vi "MAIN_save_acquisition_parameters_txt.vi"(3 "TL Array":dbl[][](array[numeric]), 4 "Global parameters":T2 {"# repetitions" min=0; "Dt (s)" min=0 step=1; "Filter list" items=["ET665lp", "zet405/488/561/640m", "None", "None", "None", "None"]}, 5 "List probe Refnum":refnum<vi>, 6 "file path":path, 7 "Data":T1, 8 "error in":errorcluster, 9 "ROI list Refnum":refnum<vi>, 10 "Laser list Refnum":refnum<vi>, 11 "Data type":string) -> (0 "error out":errorcluster)   [LabVIEW 2015]
uses:
  CONTROLS/Global parameters.ctl
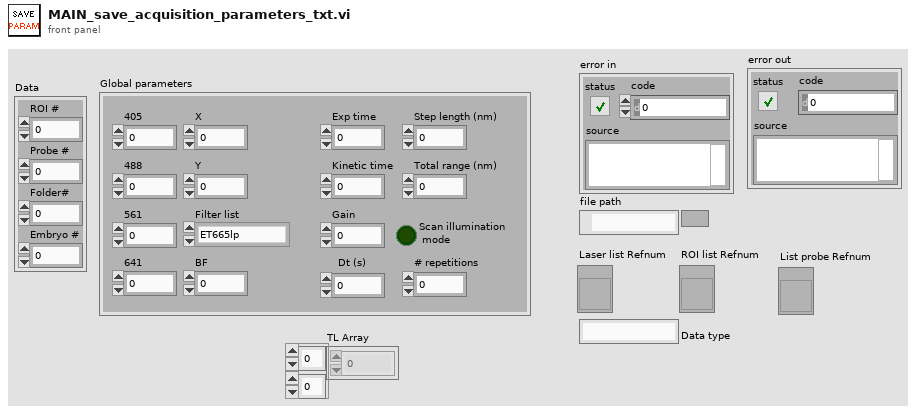
[diagram p1: front panel]
types:
  T1 = cluster{"ROI #":i32, "Probe #":i32, "Folder# ":i32, "Embryo #":i32}
  T2 = typedef "Global parameters.ctl" = cluster{"405":dbl, "488":dbl, "561":dbl, "641":dbl, "BF":dbl, "X":dbl, "Y":dbl, "Filter list":u16, "Exp time":sgl, "Kinetic time":sgl, "Gain":i32, "Step length (nm)":u32, "Total range (nm)":u32, "Scan illumination\n mode":bool, "Dt (s)":i32, "# repetitions":i32}
  T3 = enum16{"open", "replace", "create", "open or create", "replace or create", "replace or create with confirmation"}
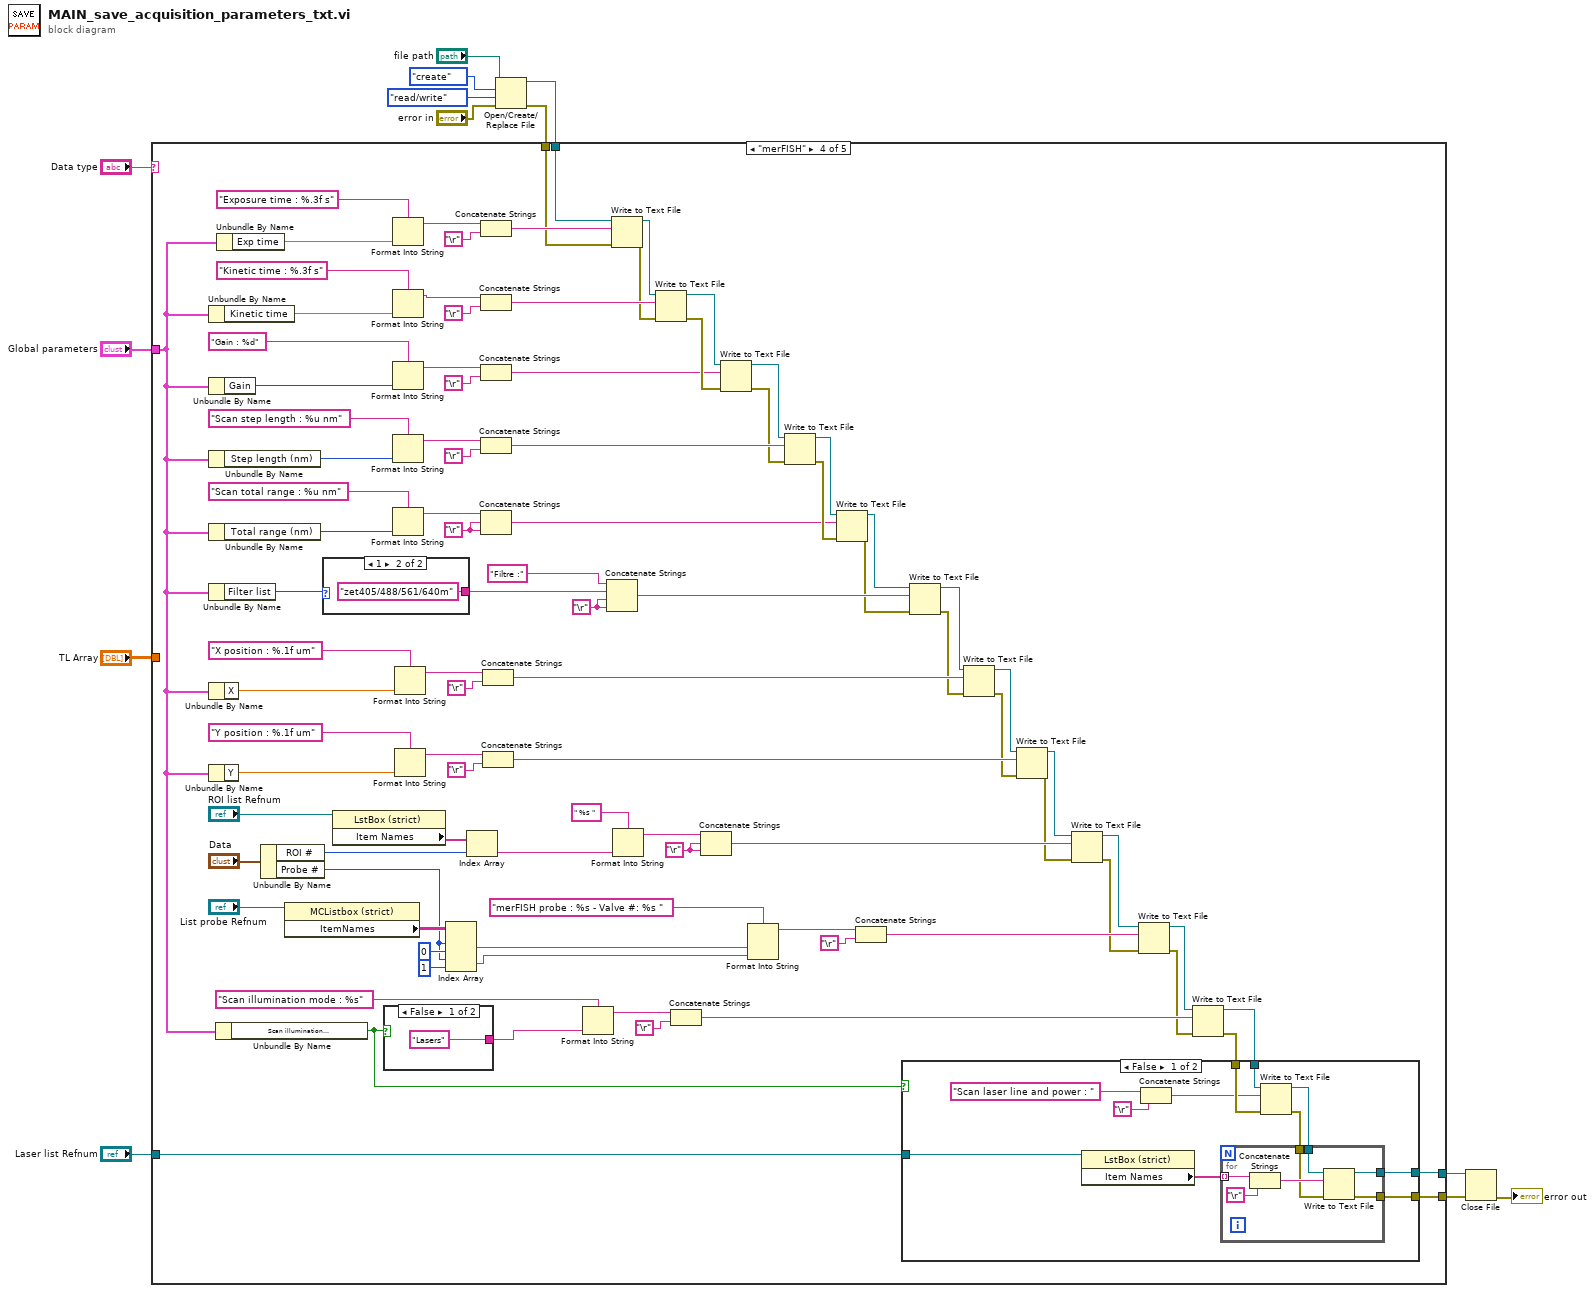
[diagram p0: block diagram]
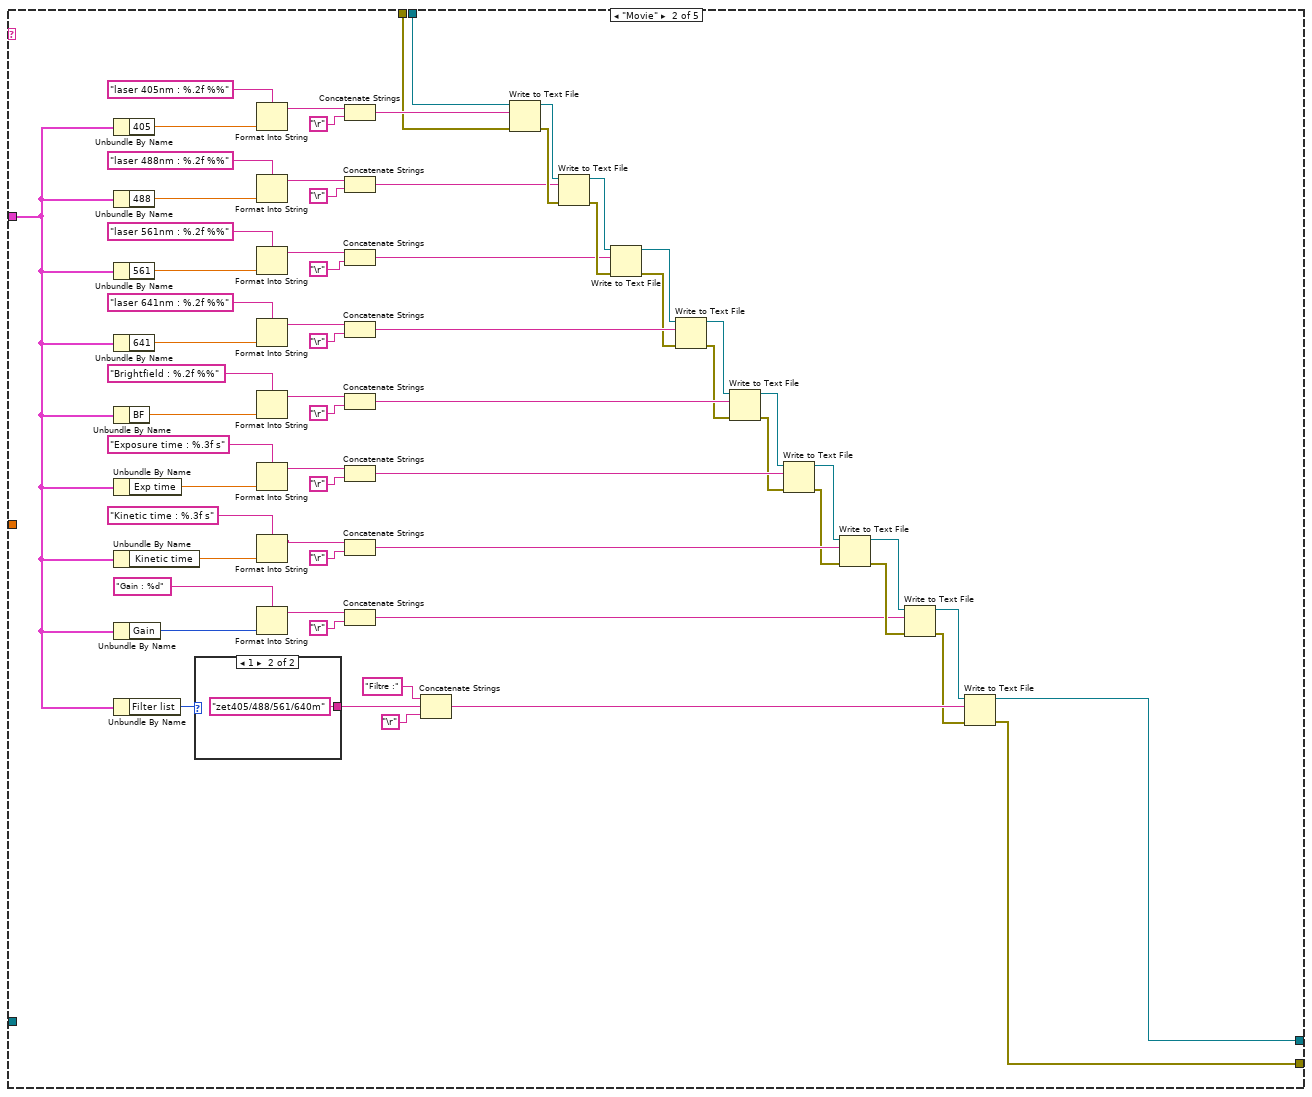
[diagram p3: hidden frame]
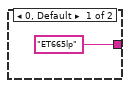
[diagram p4: hidden frame]
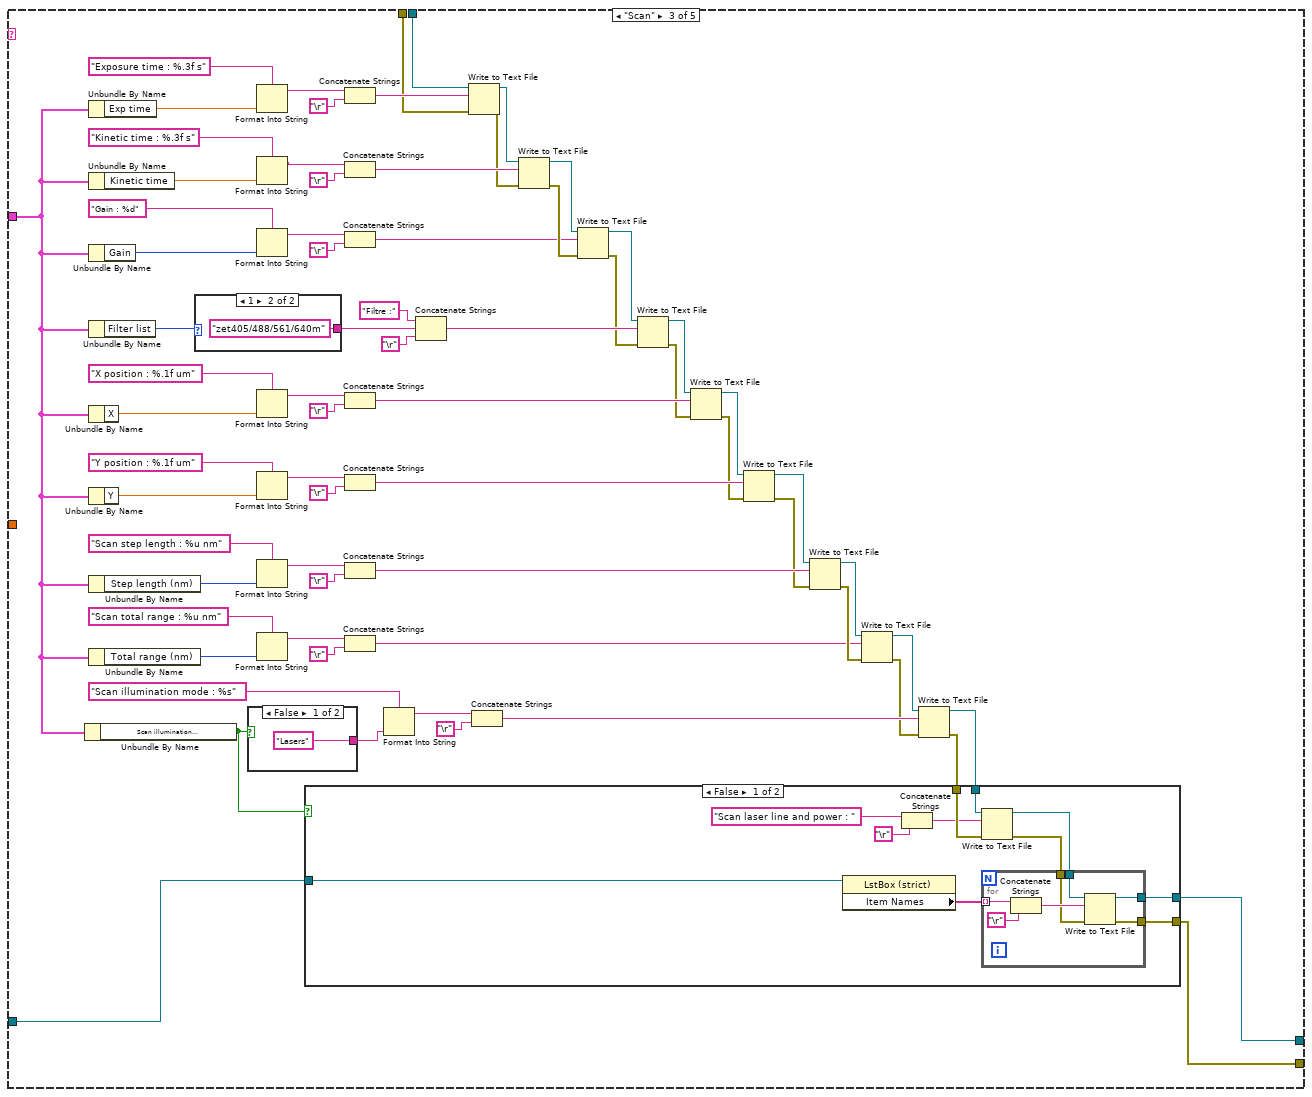
[diagram p5: hidden frame]
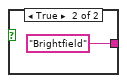
[diagram p7: hidden frame]
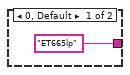
[diagram p8: hidden frame]
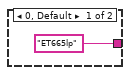
[diagram p9: hidden frame]
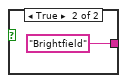
[diagram p11: hidden frame]
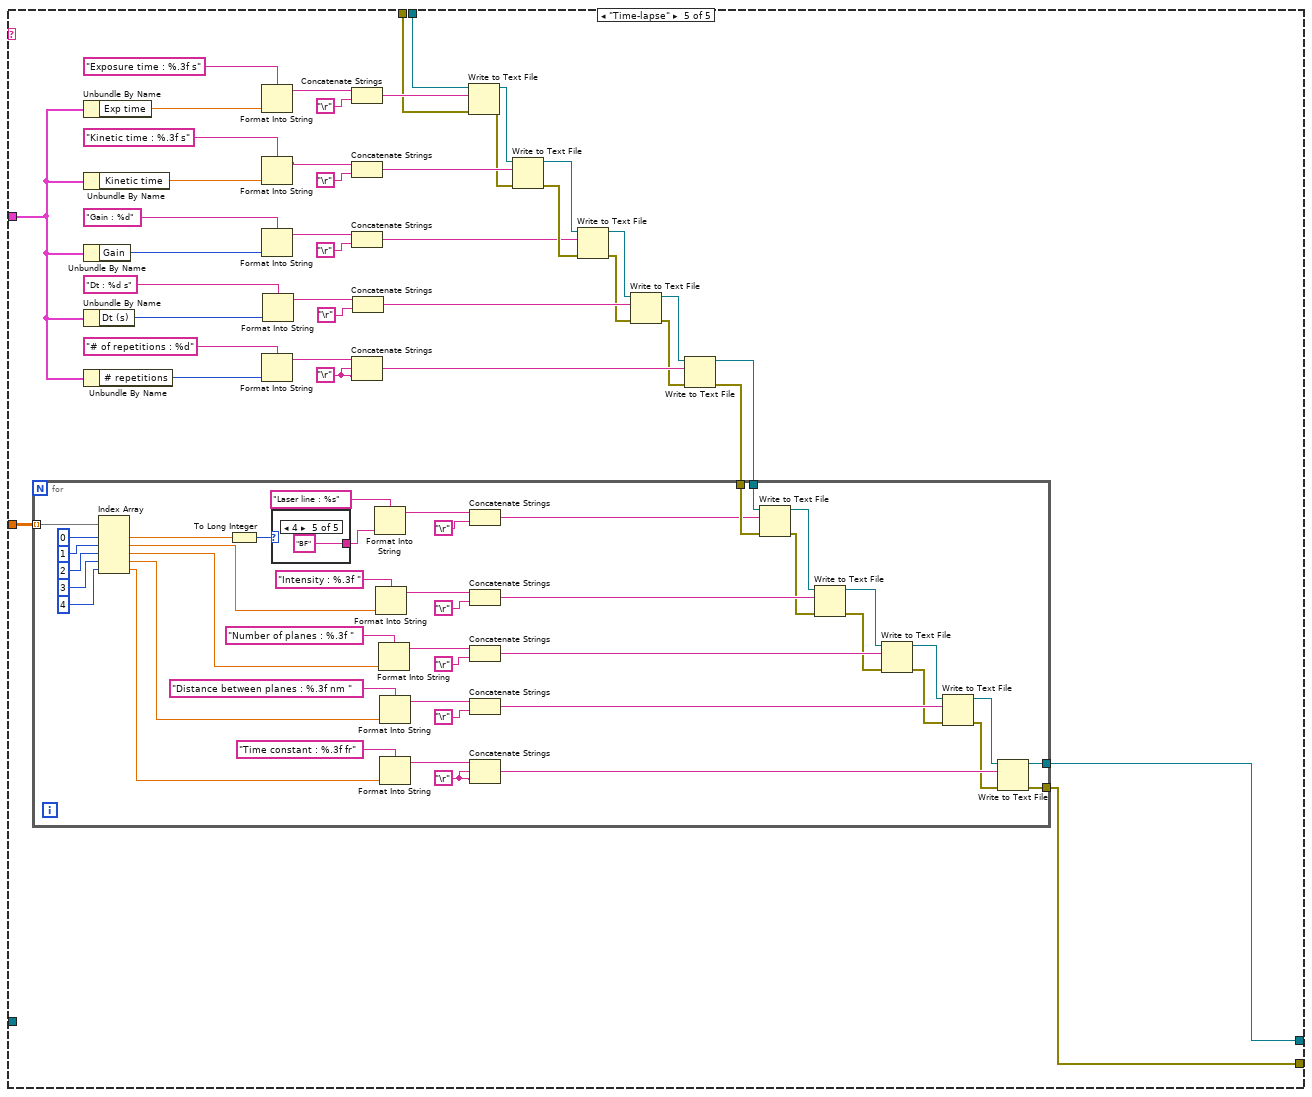
[diagram p12: hidden frame]
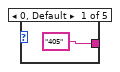
[diagram p13: hidden frame]
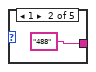
[diagram p14: hidden frame]
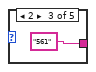
[diagram p15: hidden frame]
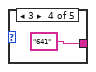
[diagram p16: hidden frame]
diagram:
  n1 = Open/Create/Replace File(file path (use dialog)="file path", error in="error in", operation (0:open)=T3."create", access (0:read/write)=enum16{"read/write", "read-only", "write-only"}."read/write") -> (refnum out=w11:refnum<file>, error out=w9:errorcluster)  [unwired: 2 in, 1 out]
  n2 = case shown="\"merFISH\"" "Data type" {
    tunnel: "Global parameters" -> [_ w19 w87 w199 w303]
    tunnel: w11 -> [w14 w16 w84 w178 w296]
    tunnel: w9 -> [w15 w17 w85 w179 w297]
    tunnel: [w15 w20 w89 w233 w316] -> w3
    tunnel: "Laser list Refnum" -> [_ _ w88 w227 _]
    tunnel: "TL Array" -> [_ _ _ _ w318]
    tunnel: [w14 w18 w86 w181 w315] -> w1
    frame "False", Default {
    }
    frame "Movie" {
      n3 = Unbundle By Name(w19) -> ("405"=w81:dbl)
      n4 = Unbundle By Name(w19) -> ("488"=w79:dbl)
      n5 = Unbundle By Name(w19) -> ("561"=w76:dbl)
      n6 = Unbundle By Name(w19) -> ("641"=w75:dbl)
      n7 = Unbundle By Name(w19) -> ("BF"=w72:dbl)
      n8 = Unbundle By Name(w19) -> ("Exp time"=w71:sgl)
      n9 = Unbundle By Name(w19) -> ("Kinetic time"=w68:sgl)
      n10 = Unbundle By Name(w19) -> ("Gain"=w67:i32)
      n11 = Unbundle By Name(w19) -> ("Filter list"=w27:u16)
      n12 = case shown="1" w27 {
        tunnel: ["ET665lp" "zet405/488/561/640m"] -> w25
        frame 0, Default {
        }
        frame 1 {
        }
      }
      n13 = Format Into String(format string="laser 405nm : %.2f %%" ("initial string"), w81) -> (resulting string=w65:string)  [unwired: 2 in, 1 out]
      n14 = Format Into String(format string="laser 488nm : %.2f %%" ("initial string"), w79) -> (resulting string=w61:string)  [unwired: 2 in, 1 out]
      n15 = Format Into String(format string="laser 561nm : %.2f %%" ("initial string"), w76) -> (resulting string=w56:string)  [unwired: 2 in, 1 out]
      n16 = Format Into String(format string="laser 641nm : %.2f %%" ("initial string"), w75) -> (resulting string=w50:string)  [unwired: 2 in, 1 out]
      n17 = Format Into String(format string="Brightfield : %.2f %%" ("initial string"), w72) -> (resulting string=w45:string)  [unwired: 2 in, 1 out]
      n18 = Format Into String(format string="Exposure time : %.3f s" ("initial string"), w71) -> (resulting string=w40:string)  [unwired: 2 in, 1 out]
      n19 = Format Into String(format string="Kinetic time : %.3f s" ("initial string"), w68) -> (resulting string=w36:string)  [unwired: 2 in, 1 out]
      n20 = Format Into String(format string="Gain : %d" ("initial string"), w67) -> (resulting string=w31:string)  [unwired: 2 in, 1 out]
      n21 = Concatenate Strings(w65, "\r") -> (w63:string)
      n22 = Concatenate Strings(w61, "\r") -> (w59:string)
      n23 = Concatenate Strings(w56, "\r") -> (w54:string)
      n24 = Concatenate Strings(w50, "\r") -> (w52:string)
      n25 = Concatenate Strings(w45, "\r") -> (w46:string)
      n26 = Concatenate Strings(w40, "\r") -> (w42:string)
      n27 = Concatenate Strings(w36, "\r") -> (w35:string)
      n28 = Concatenate Strings(w31, "\r") -> (w29:string)
      n29 = Concatenate Strings("Filtre :" ("initial string"), w25, "\r") -> (w23:string)
      n30 = Write to Text File(file (use dialog)=w16, text=w63, error in=w17) -> (refnum out=w58:refnum<file>, error out=w60:errorcluster)  [unwired: 1 in, 1 out]
      n31 = Write to Text File(file (use dialog)=w58, text=w59, error in=w60) -> (refnum out=w53:refnum<file>, error out=w55:errorcluster)  [unwired: 1 in, 1 out]
      n32 = Write to Text File(file (use dialog)=w53, text=w54, error in=w55) -> (refnum out=w48:refnum<file>, error out=w49:errorcluster)  [unwired: 1 in, 1 out]
      n33 = Write to Text File(file (use dialog)=w48, text=w52, error in=w49) -> (refnum out=w43:refnum<file>, error out=w44:errorcluster)  [unwired: 1 in, 1 out]
      n34 = Write to Text File(file (use dialog)=w43, text=w46, error in=w44) -> (refnum out=w38:refnum<file>, error out=w39:errorcluster)  [unwired: 1 in, 1 out]
      n35 = Write to Text File(file (use dialog)=w38, text=w42, error in=w39) -> (refnum out=w33:refnum<file>, error out=w34:errorcluster)  [unwired: 1 in, 1 out]
      n36 = Write to Text File(file (use dialog)=w33, text=w35, error in=w34) -> (refnum out=w28:refnum<file>, error out=w30:errorcluster)  [unwired: 1 in, 1 out]
      n37 = Write to Text File(file (use dialog)=w28, text=w29, error in=w30) -> (refnum out=w21:refnum<file>, error out=w22:errorcluster)  [unwired: 1 in, 1 out]
      n38 = Write to Text File(file (use dialog)=w21, text=w23, error in=w22) -> (refnum out=w18:refnum<file>, error out=w20:errorcluster)  [unwired: 1 in, 1 out]
    }
    frame "Scan" {
      n39 = Unbundle By Name(w87) -> ("Scan illumination\n mode"=w92:bool)
      n40 = Unbundle By Name(w87) -> ("Exp time"=w153:sgl)
      n41 = Unbundle By Name(w87) -> ("Kinetic time"=w150:sgl)
      n42 = Unbundle By Name(w87) -> ("Gain"=w149:i32)
      n43 = Unbundle By Name(w87) -> ("Filter list"=w134:u16)
      n44 = Unbundle By Name(w87) -> ("X"=w123:dbl)
      n45 = Unbundle By Name(w87) -> ("Y"=w120:dbl)
      n46 = Unbundle By Name(w87) -> ("Step length (nm)"=w113:u32)
      n47 = Unbundle By Name(w87) -> ("Total range (nm)"=w106:u32)
      n48 = case shown="1" w134 {
        tunnel: ["ET665lp" "zet405/488/561/640m"] -> w132
        frame 0, Default {
        }
        frame 1 {
        }
      }
      n49 = case shown="False" w92 {
        tunnel: ["Lasers" ("initial string") "Brightfield" ("initial string")] -> w95
        frame False {
        }
        frame True {
        }
      }
      n50 = Format Into String(format string="Exposure time : %.3f s" ("initial string"), w153) -> (resulting string=w145:string)  [unwired: 2 in, 1 out]
      n51 = Format Into String(format string="Kinetic time : %.3f s" ("initial string"), w150) -> (resulting string=w143:string)  [unwired: 2 in, 1 out]
      n52 = Format Into String(format string="Gain : %d" ("initial string"), w149) -> (resulting string=w138:string)  [unwired: 2 in, 1 out]
      n53 = Format Into String(format string="X position : %.1f um" ("initial string"), w123) -> (resulting string=w126:string)  [unwired: 2 in, 1 out]
      n54 = Format Into String(format string="Y position : %.1f um" ("initial string"), w120) -> (resulting string=w117:string)  [unwired: 2 in, 1 out]
      n55 = Format Into String(format string="Scan step length : %u nm" ("initial string"), w113) -> (resulting string=w110:string)  [unwired: 2 in, 1 out]
      n56 = Format Into String(format string="Scan total range : %u nm" ("initial string"), w106) -> (resulting string=w108:string)  [unwired: 2 in, 1 out]
      n57 = Concatenate Strings(w145, "\r") -> (w147:string)
      n58 = Concatenate Strings(w143, "\r") -> (w142:string)
      n59 = Concatenate Strings(w138, "\r") -> (w136:string)
      n60 = Concatenate Strings(w126, "\r") -> (w127:string)
      n61 = Concatenate Strings(w117, "\r") -> (w116:string)
      n62 = Concatenate Strings(w110, "\r") -> (w109:string)
      n63 = Concatenate Strings(w108, "\r") -> (w104:string)
      n64 = Format Into String(format string="Scan illumination mode : %s" ("initial string"), w95) -> (resulting string=w96:string)  [unwired: 2 in, 1 out]
      n65 = Concatenate Strings("Filtre :" ("initial string"), w132, "\r") -> (w130:string)
      n66 = Write to Text File(file (use dialog)=w84, text=w147, error in=w85) -> (refnum out=w140:refnum<file>, error out=w141:errorcluster)  [unwired: 1 in, 1 out]
      n67 = Concatenate Strings(w96, "\r") -> (w98:string)
      n68 = Write to Text File(file (use dialog)=w140, text=w142, error in=w141) -> (refnum out=w135:refnum<file>, error out=w137:errorcluster)  [unwired: 1 in, 1 out]
      n69 = Write to Text File(file (use dialog)=w135, text=w136, error in=w137) -> (refnum out=w128:refnum<file>, error out=w129:errorcluster)  [unwired: 1 in, 1 out]
      n70 = Write to Text File(file (use dialog)=w128, text=w130, error in=w129) -> (refnum out=w121:refnum<file>, error out=w122:errorcluster)  [unwired: 1 in, 1 out]
      n71 = Write to Text File(file (use dialog)=w121, text=w127, error in=w122) -> (refnum out=w114:refnum<file>, error out=w115:errorcluster)  [unwired: 1 in, 1 out]
      n72 = Write to Text File(file (use dialog)=w114, text=w116, error in=w115) -> (refnum out=w100:refnum<file>, error out=w101:errorcluster)  [unwired: 1 in, 1 out]
      n73 = Write to Text File(file (use dialog)=w100, text=w109, error in=w101) -> (refnum out=w103:refnum<file>, error out=w105:errorcluster)  [unwired: 1 in, 1 out]
      n74 = Write to Text File(file (use dialog)=w103, text=w104, error in=w105) -> (refnum out=w93:refnum<file>, error out=w94:errorcluster)  [unwired: 1 in, 1 out]
      n75 = Write to Text File(file (use dialog)=w93, text=w98, error in=w94) -> (refnum out=w90:refnum<file>, error out=w91:errorcluster)  [unwired: 1 in, 1 out]
      n76 = case shown="False" w92 {
        tunnel: w91 -> [w164 w173]
        tunnel: w90 -> [w163 w172]
        tunnel: [w157 w173] -> w89
        tunnel: w88 -> [w155 _]
        tunnel: [w154 w172] -> w86
        frame False {
          n77 = property class="LstBox (strict)"(reference=w155) -> ("Item Names"=w160:string[])  [unwired: 1 in, 2 out]
          n78 = Concatenate Strings("Scan laser line and power : " ("initial string"), "\r") -> (w162:string)
          n79 = Write to Text File(file (use dialog)=w163, text=w162, error in=w164) -> (refnum out=w159:refnum<file>, error out=w158:errorcluster)  [unwired: 1 in, 1 out]
          n80 = for {
            tunnel: w160 -> [w171] mode=indexing
            tunnel: w159 -> [w168]
            tunnel: w158 -> [w167]
            tunnel: [w166] -> w157
            tunnel: [w165] -> w154
            n81 = Concatenate Strings(w171, "\r") -> (w169:string)
            n82 = Write to Text File(file (use dialog)=w168, text=w169, error in=w167) -> (refnum out=w165:refnum<file>, error out=w166:errorcluster)  [unwired: 1 in, 1 out]
          }
        }
        frame True {
        }
      }
    }
    frame "merFISH" {
      w205 = "\r"
      w225 = "\r"
      w226 = "\r"
      n83 = Unbundle By Name(w199) -> ("Kinetic time"=w268:sgl)
      n84 = Unbundle By Name(w199) -> ("Gain"=w267:i32)
      n85 = Unbundle By Name(w199) -> ("Step length (nm)"=w252:u32)
      n86 = Unbundle By Name(w199) -> ("Total range (nm)"=w246:u32)
      n87 = Unbundle By Name(w199) -> ("Filter list"=w208:u16)
      n88 = Unbundle By Name(w199) -> ("X"=w220:dbl)
      n89 = Unbundle By Name(w199) -> ("Y"=w219:dbl)
      n90 = Unbundle By Name(w199) -> ("Scan illumination\n mode"=w236:bool)
      n91 = Unbundle By Name(w199) -> ("Exp time"=w271:sgl)
      n92 = Unbundle By Name("Data") -> ("ROI #"=w197:i32, "Probe #"=w184:i32)
      n93 = property class="MCListbox (strict)"(reference="List probe Refnum") -> ("ItemNames"=w195:string[][])  [unwired: 1 in, 2 out]
      n94 = case shown="1" w208 {
        tunnel: ["ET665lp" "zet405/488/561/640m"] -> w206
        frame 0, Default {
        }
        frame 1 {
        }
      }
      n95 = property class="LstBox (strict)"(reference="ROI list Refnum") -> ("Item Names"=w232:string[])  [unwired: 1 in, 2 out]
      n96 = case shown="False" w236 {
        tunnel: ["Lasers" ("initial string") "Brightfield" ("initial string")] -> w237
        frame False {
        }
        frame True {
        }
      }
      n97 = Format Into String(format string="Exposure time : %.3f s" ("initial string"), w271) -> (resulting string=w263:string)  [unwired: 2 in, 1 out]
      n98 = Format Into String(format string="Kinetic time : %.3f s" ("initial string"), w268) -> (resulting string=w261:string)  [unwired: 2 in, 1 out]
      n99 = Format Into String(format string="Gain : %d" ("initial string"), w267) -> (resulting string=w256:string)  [unwired: 2 in, 1 out]
      n100 = Format Into String(format string="Scan step length : %u nm" ("initial string"), w252) -> (resulting string=w249:string)  [unwired: 2 in, 1 out]
      n101 = Format Into String(format string="Scan total range : %u nm" ("initial string"), w246) -> (resulting string=w247:string)  [unwired: 2 in, 1 out]
      n102 = Format Into String(format string="X position : %.1f um" ("initial string"), w220) -> (resulting string=w223:string)  [unwired: 2 in, 1 out]
      n103 = Format Into String(format string="Y position : %.1f um" ("initial string"), w219) -> (resulting string=w216:string)  [unwired: 2 in, 1 out]
      n104 = Index Array(array=w195, index (row) #1=w184, index (col) #1=0 ("disabled index (col)"), index (row) #2=w184, index (col) #2=1 ("disabled index (col)")) -> (element #1=w190:string, element #2=w182:string)
      n105 = Index Array(array=w232, index=w197) -> (element=w229:string)
      n106 = Concatenate Strings(w263, "\r") -> (w265:string)
      n107 = Concatenate Strings(w261, "\r") -> (w260:string)
      n108 = Concatenate Strings(w256, "\r") -> (w254:string)
      n109 = Concatenate Strings(w249, "\r") -> (w248:string)
      n110 = Concatenate Strings(w247, w226, w226) -> (w244:string)
      n111 = Concatenate Strings(w223, "\r") -> (w224:string)
      n112 = Concatenate Strings(w216, "\r") -> (w215:string)
      n113 = Format Into String(format string="Scan illumination mode : %s" ("initial string"), w237) -> (resulting string=w238:string)  [unwired: 2 in, 1 out]
      n114 = Concatenate Strings("Filtre :" ("initial string"), w206, w205, w205) -> (w204:string)
      n115 = Write to Text File(file (use dialog)=w178, text=w265, error in=w179) -> (refnum out=w258:refnum<file>, error out=w259:errorcluster)  [unwired: 1 in, 1 out]
      n116 = Format Into String(format string=" %s " ("initial string"), w229) -> (resulting string=w230:string)  [unwired: 2 in, 1 out]
      n117 = Write to Text File(file (use dialog)=w258, text=w260, error in=w259) -> (refnum out=w253:refnum<file>, error out=w255:errorcluster)  [unwired: 1 in, 1 out]
      n118 = Concatenate Strings(w238, "\r") -> (w240:string)
      n119 = Concatenate Strings(w230, w225, w225) -> (w228:string)
      n120 = Write to Text File(file (use dialog)=w253, text=w254, error in=w255) -> (refnum out=w209:refnum<file>, error out=w210:errorcluster)  [unwired: 1 in, 1 out]
      n121 = Format Into String(format string="merFISH probe : %s - Valve #: %s " ("initial string"), w190, w182) -> (resulting string=w192:string)  [unwired: 2 in, 1 out]
      n122 = Write to Text File(file (use dialog)=w209, text=w248, error in=w210) -> (refnum out=w243:refnum<file>, error out=w245:errorcluster)  [unwired: 1 in, 1 out]
      n123 = Write to Text File(file (use dialog)=w243, text=w244, error in=w245) -> (refnum out=w201:refnum<file>, error out=w200:errorcluster)  [unwired: 1 in, 1 out]
      n124 = Concatenate Strings(w192, "\r") -> (w187:string)
      n125 = Write to Text File(file (use dialog)=w201, text=w204, error in=w200) -> (refnum out=w202:refnum<file>, error out=w203:errorcluster)  [unwired: 1 in, 1 out]
      n126 = Write to Text File(file (use dialog)=w202, text=w224, error in=w203) -> (refnum out=w213:refnum<file>, error out=w214:errorcluster)  [unwired: 1 in, 1 out]
      n127 = Write to Text File(file (use dialog)=w213, text=w215, error in=w214) -> (refnum out=w212:refnum<file>, error out=w211:errorcluster)  [unwired: 1 in, 1 out]
      n128 = Write to Text File(file (use dialog)=w212, text=w228, error in=w211) -> (refnum out=w189:refnum<file>, error out=w186:errorcluster)  [unwired: 1 in, 1 out]
      n129 = Write to Text File(file (use dialog)=w189, text=w187, error in=w186) -> (refnum out=w188:refnum<file>, error out=w185:errorcluster)  [unwired: 1 in, 1 out]
      n130 = Write to Text File(file (use dialog)=w188, text=w240, error in=w185) -> (refnum out=w234:refnum<file>, error out=w235:errorcluster)  [unwired: 1 in, 1 out]
      n131 = case shown="False" w236 {
        tunnel: w235 -> [w284 w293]
        tunnel: w234 -> [w283 w292]
        tunnel: [w277 w293] -> w233
        tunnel: w227 -> [w275 _]
        tunnel: [w274 w292] -> w181
        frame False {
          n132 = property class="LstBox (strict)"(reference=w275) -> ("Item Names"=w280:string[])  [unwired: 1 in, 2 out]
          n133 = Concatenate Strings("Scan laser line and power : " ("initial string"), "\r") -> (w282:string)
          n134 = Write to Text File(file (use dialog)=w283, text=w282, error in=w284) -> (refnum out=w279:refnum<file>, error out=w278:errorcluster)  [unwired: 1 in, 1 out]
          n135 = for {
            tunnel: w280 -> [w291] mode=indexing
            tunnel: w279 -> [w288]
            tunnel: w278 -> [w287]
            tunnel: [w286] -> w277
            tunnel: [w285] -> w274
            n136 = Concatenate Strings(w291, "\r") -> (w289:string)
            n137 = Write to Text File(file (use dialog)=w288, text=w289, error in=w287) -> (refnum out=w285:refnum<file>, error out=w286:errorcluster)  [unwired: 1 in, 1 out]
          }
        }
        frame True {
        }
      }
    }
    frame "Time-lapse" {
      w298 = "\r"
      n138 = Unbundle By Name(w303) -> ("Exp time"=w336:sgl)
      n139 = Unbundle By Name(w303) -> ("Kinetic time"=w333:sgl)
      n140 = Unbundle By Name(w303) -> ("Gain"=w332:i32)
      n141 = Unbundle By Name(w303) -> ("Dt (s)"=w311:i32)
      n142 = Unbundle By Name(w303) -> ("# repetitions"=w306:i32)
      n143 = Format Into String(format string="Exposure time : %.3f s" ("initial string"), w336) -> (resulting string=w328:string)  [unwired: 2 in, 1 out]
      n144 = Format Into String(format string="Kinetic time : %.3f s" ("initial string"), w333) -> (resulting string=w326:string)  [unwired: 2 in, 1 out]
      n145 = Format Into String(format string="Gain : %d" ("initial string"), w332) -> (resulting string=w322:string)  [unwired: 2 in, 1 out]
      n146 = Format Into String(format string="# of repetitions : %d" ("initial string"), w306) -> (resulting string=w305:string)  [unwired: 2 in, 1 out]
      n147 = Format Into String(format string="Dt : %d s" ("initial string"), w311) -> (resulting string=w312:string)  [unwired: 2 in, 1 out]
      n148 = Concatenate Strings(w328, "\r") -> (w330:string)
      n149 = Concatenate Strings(w326, "\r") -> (w325:string)
      n150 = Concatenate Strings(w322, "\r") -> (w320:string)
      n151 = Concatenate Strings(w305, w298, w298) -> (w304:string)
      n152 = Concatenate Strings(w312, "\r") -> (w313:string)
      n153 = Write to Text File(file (use dialog)=w296, text=w330, error in=w297) -> (refnum out=w323:refnum<file>, error out=w324:errorcluster)  [unwired: 1 in, 1 out]
      n154 = Write to Text File(file (use dialog)=w323, text=w325, error in=w324) -> (refnum out=w319:refnum<file>, error out=w321:errorcluster)  [unwired: 1 in, 1 out]
      n155 = Write to Text File(file (use dialog)=w319, text=w320, error in=w321) -> (refnum out=w308:refnum<file>, error out=w309:errorcluster)  [unwired: 1 in, 1 out]
      n156 = Write to Text File(file (use dialog)=w308, text=w313, error in=w309) -> (refnum out=w301:refnum<file>, error out=w302:errorcluster)  [unwired: 1 in, 1 out]
      n157 = Write to Text File(file (use dialog)=w301, text=w304, error in=w302) -> (refnum out=w299:refnum<file>, error out=w300:errorcluster)  [unwired: 1 in, 1 out]
      n158 = for {
        tunnel: w318 -> [w378] mode=indexing
        tunnel: w300 -> [w375]
        tunnel: w299 -> [w376]
        tunnel: [w338] -> w316
        tunnel: [w337] -> w315
        w339 = "\r"
        n159 = Index Array(array=w378, index #1=0 ("index"), index #2=1 ("index"), index #3=2 ("index"), index #4=3 ("index"), index #5=4 ("index")) -> (element #1=w370:dbl, element #2=w366:dbl, element #3=w355:dbl, element #4=w349:dbl, element #5=w344:dbl)
        n160 = To Long Integer(number=w370) -> (32bit integer=w369:i32)
        n161 = case shown="4" w369 {
          tunnel: ["405" "488" "561" "641" "BF"] -> w368
          frame 0, Default {
          }
          frame 1 {
          }
          frame 2 {
          }
          frame 3 {
          }
          frame 4 {
          }
        }
        n162 = Format Into String(format string="Laser line : %s" ("initial string"), w368) -> (resulting string=w381:string)  [unwired: 2 in, 1 out]
        n163 = Format Into String(format string="Intensity : %.3f " ("initial string"), w366) -> (resulting string=w371:string)  [unwired: 2 in, 1 out]
        n164 = Format Into String(format string="Number of planes : %.3f " ("initial string"), w355) -> (resulting string=w361:string)  [unwired: 2 in, 1 out]
        n165 = Format Into String(format string="Distance between planes : %.3f nm " ("initial string"), w349) -> (resulting string=w351:string)  [unwired: 2 in, 1 out]
        n166 = Format Into String(format string="Time constant : %.3f fr" ("initial string"), w344) -> (resulting string=w345:string)  [unwired: 2 in, 1 out]
        n167 = Concatenate Strings(w381, "\r") -> (w374:string)
        n168 = Concatenate Strings(w371, "\r") -> (w365:string)
        n169 = Concatenate Strings(w361, "\r") -> (w362:string)
        n170 = Concatenate Strings(w351, "\r") -> (w350:string)
        n171 = Concatenate Strings(w345, w339, w339) -> (w342:string)
        n172 = Write to Text File(file (use dialog)=w376, text=w374, error in=w375) -> (refnum out=w363:refnum<file>, error out=w364:errorcluster)  [unwired: 1 in, 1 out]
        n173 = Write to Text File(file (use dialog)=w363, text=w365, error in=w364) -> (refnum out=w357:refnum<file>, error out=w358:errorcluster)  [unwired: 1 in, 1 out]
        n174 = Write to Text File(file (use dialog)=w357, text=w362, error in=w358) -> (refnum out=w348:refnum<file>, error out=w347:errorcluster)  [unwired: 1 in, 1 out]
        n175 = Write to Text File(file (use dialog)=w348, text=w350, error in=w347) -> (refnum out=w340:refnum<file>, error out=w341:errorcluster)  [unwired: 1 in, 1 out]
        n176 = Write to Text File(file (use dialog)=w340, text=w342, error in=w341) -> (refnum out=w337:refnum<file>, error out=w338:errorcluster)  [unwired: 1 in, 1 out]
      }
    }
  }
  n177 = Close File(refnum=w1, error in=w3) -> (error out=→"error out":errorcluster)  [unwired: 1 out]
